vi "6.1.1.-Lógica Difusa Motor.vi"() -> (3 "Posicion":dbl(knob), 11 "Tensión":dbl(slide) scale=-12.0..12.0)   [LabVIEW 2020]
uses:
  <vilib>/addons/Fuzzy Logic/FL Fuzzy Controller (SISO).vi
  <vilib>/addons/Fuzzy Logic/NI_Fuzzy_Logic_API.lvlib
panel:
  out "XY Graph":cluster{i32[], dbl[]}(graph)
  out "Array":dbl[](array[numeric])
  in  "stop":bool
  in  "Set Point":dbl(slide) scale=0.0..360.0
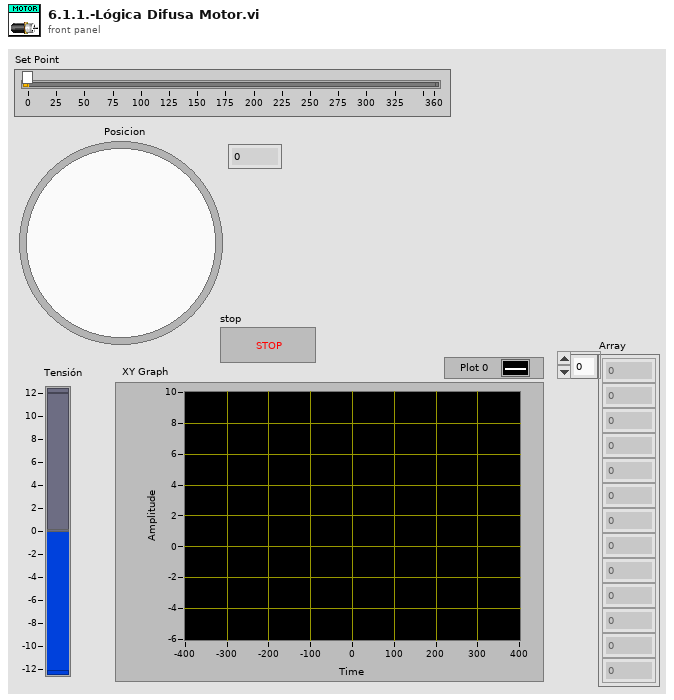
[diagram p1: front panel]
types:
  T1 = typedef "NI_Fuzzy_Logic_API.lvlib/FL System.ctl" = cluster{"input variables":T2[], "output variables":T2[], "rules":T5[], "defuzzification method":T11, "description":string, "user MF interpolating polynomials":T12[]}
  T2 = typedef "NI_Fuzzy_Logic_API.lvlib/FL Variable.ctl" = cluster{"name":string, "range":dbl[], "MFs":T3[]}
  T3 = typedef "NI_Fuzzy_Logic_API.lvlib/FL Membership Function.ctl" = cluster{"name":string, "shape":T4, "points":dbl[], "color":u32, "user-defined shape index":i32}
  T4 = typedef "NI_Fuzzy_Logic_API.lvlib/FL Membership Function Shape.ctl" = u16
  T5 = typedef "NI_Fuzzy_Logic_API.lvlib/FL Rule.ctl" = cluster{"antecedents":T6[], "antecedent connective":T8, "consequents":T9[], "consequent implication":T10, "degree of support":dbl}
  T6 = typedef "NI_Fuzzy_Logic_API.lvlib/FL Antecedent.ctl" = cluster{"Var Index":i32, "MF Index":i32, "Cond":T7}
  T7 = typedef "NI_Fuzzy_Logic_API.lvlib/FL Modifier.ctl" = u16
  T8 = typedef "NI_Fuzzy_Logic_API.lvlib/FL Antecedent Connective.ctl" = u16
  T9 = typedef "NI_Fuzzy_Logic_API.lvlib/FL Consequent.ctl" = cluster{"Var Index":i32, "MF Index":i32, "Cond":T7}
  T10 = typedef "NI_Fuzzy_Logic_API.lvlib/FL Consequent Implication.ctl" = u16
  T11 = typedef "NI_Fuzzy_Logic_API.lvlib/FL Defuzzification.ctl" = u16
  T12 = typedef "NI_Fuzzy_Logic_API.lvlib/FL Interpolating polynomials.ctl" = cluster{"X":dbl[], "Y":dbl[], "Y(x) coeff":dbl[][], "X(y) coeff":dbl[][], "Area(y) coeff":dbl[][], "coa_x(y) coeff":dbl[][]}
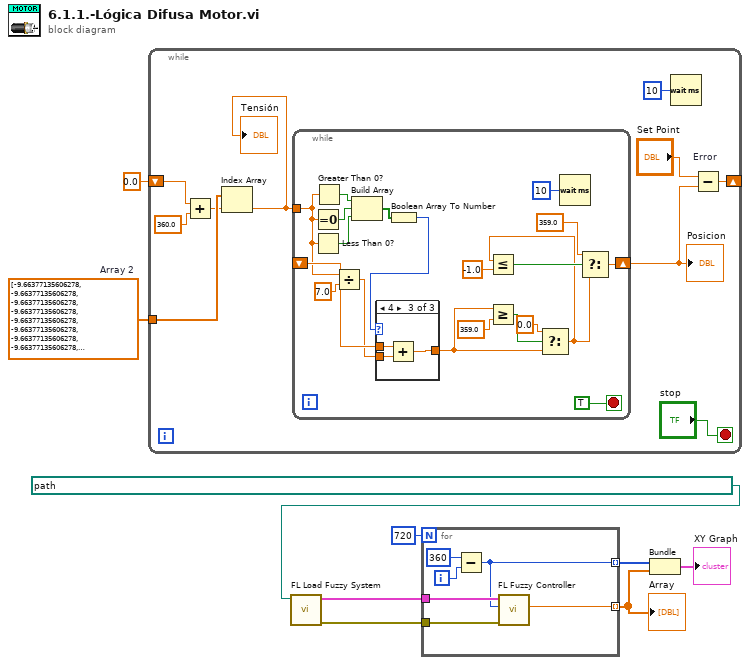
[diagram p0: block diagram]
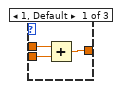
[diagram p2: hidden frame]
diagram:
  w1 = dbl[] [-9.66377135606278, -9.66377135606278, -9.66377135606278, -9.66377135606278, -9.66377135606278, -9.66377135606278, -9.66377135606278, -9.66377135606278, -9.66377135606278, -9.66377135606278, -9.66377135606278, -9.66377135606278, -9.66377135606278, -9.66377135606278, -9.66377135606278, -9.66377135606278, -9.66377135606278, -9.66377135606278, -9.66377135606278, -9.66377135606278, -9.66377135606278, -9.66377135606278, -9.66377135606278, -9.66377135606278, -9.66377135606278, -9.66377135606278, -9.66377135606278, -9.66377135606278, -9.66377135606278, -9.66377135606278, -9.66377135606278, -9.66377135606278, -9.66377135606278, -9.66377135606278, -9.66377135606278, -9.66377135606278, -9.66377135606278, -9.66377135606278, -9.66377135606278, -9.66377135606278, -9.66377135606278, -9.66377135606278, -9.66377135606278, -9.66377135606278, -9.66377135606278, -9.66377135606278, -9.66377135606278, -9.66377135606278, -9.66377135606278, -9.66377135606278, -9.66377135606278, -9.66377135606278, -9.66377135606278, -9.66377135606278, -9.66377135606278, -9.66377135606278, -9.66377135606278, -9.66377135606278, -9.66377135606278, -9.66377135606278, -9.66377135606278, -9.602567611575033, -9.541862924617375, -9.481651215975328, -9.421926504772852, -9.362682906491901, -9.303914631039657, -9.244328181919316, -9.187821091365203, -9.133216921575809, -9.079043687583988, -9.025296308026498, -8.971969781116245, -8.91905918309065, -8.866559666696107, -8.814466459707706, -8.76277486348314, -8.711480251549936, -8.66057806822514, -8.610063827266517, -8.559933110554525, -8.510181566804137, -8.46074884357682, -8.418094863909172, -8.375889018091348, -8.33385061736725, -8.291978667241288, -8.250272181077706, -8.208730180023073, -8.167351692929728, -8.126135756280064, -8.08458400446258, -8.042461828178011, -8.00057677537656, -7.95892684937627, -7.917510075849662, -7.876324502511783, -7.836119326659839, -7.79819112131189, -7.760440752628416, -7.722866972781734, -7.685468545591136, -7.648244246387266, -7.611192861878472, -7.574313190018964, -7.537604039878832, -7.5010443555021755, -7.464413266940578, -7.4279199209420534, -7.391563542041992, -7.355343360585824, -7.319258612674724, -7.285949116533284, -7.254699798339329, -7.223515170326685, -7.192395031827329, -7.161317190840123, -7.130325267582253, -7.099422687499635, -7.068609064812042, -7.037884015957109, -7.007247159574394, -6.976698116489636, -6.9462365096990695, -6.91586196435395, -6.88557410774515, -6.855372569287947, -6.8269062701543985, -6.7987291960853815, -6.77060930354623, -6.742546418650207, -6.714119548633666, -6.685283733960341, -6.656408950727237, -6.627522459838097, -6.598624254170943, -6.569714326598021, -6.540792669985794, -6.511859277194934, -6.482914141080324, -6.4539572544910335, -6.4255452155999135, -6.399570969318972, -6.373543875051162, -6.347463771343066, -6.321330496082931, -6.295143886497309, -6.268903779147681, -6.242610009927052, -6.216262414056531, -6.189701785954419, -6.162867037973021, -6.135932903288173, -6.10889882873411, -6.081764257032361, -6.054528626753464, -6.027768904888585, -6.0014956107977575, -5.976187022973889, -5.9510616641367875, -5.925862874705745, -5.900590332300716, -5.8752437126517645, -5.8498226895852135, -5.824326935009648, -5.79875611890179, -5.773109909292277, -5.747387972251279, -5.721574419432044, -5.695518359202395, -5.669362850943312, -5.644440395152999, -5.619727133509676, -5.594876515472104, -5.569887392708088, -5.544758604049223, -5.519973566001828, -5.495685899353129, -5.471282522457748, -5.446762606448659, -5.422125314523331, -5.397369801848523, -5.372495215463717, -5.347500694183157, -5.32238536849646, -5.29719932379442, -5.272328422653832, -5.247066777713917, -5.221525696016304, -5.195790676804522, -5.169859502762561, -5.143729922643894, -5.11739965061997, -5.0908663656136115, -5.064355820327918, -5.040639459585903, -5.016781897703681, -4.992781869903006, -4.968638096255104, -4.944349281453124, -4.920015121091849, -4.8956488914145195, -4.871089069614369, -4.846333339326462, -4.82137934708358, -4.796166136073796, -4.770627065319108, -4.744856356126937, -4.718850842712282, -4.692607301337395, -4.666122448979593, -4.666122448979593, -4.666122448979593, -4.666122448979593, -4.666122448979593, -4.666122448979593, -4.665974085361705, -4.665743113875069, -4.665511918544546, -4.6652804990445755, -4.665048855048962, -4.664823742717059, -4.664602732085556, -4.664381075696181, -4.664158770714593, -4.663935814289835, -4.663712203554218, -4.663487935623198, -4.663263007595254, -4.6630374165517505, -4.662811159556827, -4.662584233657263, -4.6623566358823485, -4.662128363243756, -4.661634601556013, -4.660440470721498, -4.65946207826866, -4.658503151845306, -4.657538463367321, -4.65656796074313, -4.655591591251354, -4.654609301531252, -4.65362103757302, -4.652626744707875, -4.651626367597976, -4.650619850226163, -4.649607135885501, -4.648588167168621, -4.647562885956887, -4.646531233409329, -4.645699289179396, -4.645668560719857, -4.645637574666107, -4.644900326948918, -4.644084328893788, -4.643260525293575, -4.642428803612462, -4.641589049140895, -4.640741144942827, -4.639884971801439, -4.639020408163266, -4.638147330080661, -4.637265611152561, -4.6363751224634795, -4.63547573252067, -4.634980573065503, -4.6348790662002655, -4.634776413157728, -4.63467259441436, -4.634567590000691, -4.6344613794885055, -4.633117424753972, -4.630697548591472, -4.628243632472906, -4.625754953059972, -4.623230766373886, -4.620670307053868, -4.618072787583446, -4.615437397482888, -4.612763302466092, -4.611980173972492, -4.6116221714488965, -4.611257874415769, -4.610887115392786, -4.610509720904837, -4.610125511211395, -4.609734300021062, -4.609335894190391, -4.608930093405926, -4.608227230255004, -4.606117170096181, -4.603963880942782, -4.601766020591362, -4.59952219069252, -4.597437413307896, -4.596803168782329, -4.59615429362253, -4.595490275676275, -4.594810578604951, -4.594114640438743, -4.593401872027007, -4.59267165537482, -4.591923341855887, -4.591156250290884, -4.590369664879315, -4.589562832971661, -4.588734962667249, -4.587885220221753, -4.582953994092828, -4.578969620421459, -4.5776863654930455, -4.57635787555434, -4.574981715877343, -4.573555273812931, -4.572075742236131, -4.570540101107925, -4.568945096898777, -4.567287219578867, -4.565562676832542, -4.563767365098355, -4.56189683696917, -4.559946264407187, -4.557910397133364, -4.555783515436167, -4.556357795824015, -4.557996462536207, -4.557859524402199, -4.555272430381818, -4.55254080072598, -4.549652175001101, -4.546592618109409, -4.543346495483677, -4.539896205864125, -4.5362218620166965, -4.532300907163601, -4.528107651499963, -4.523612708673419, -4.518782306096311, -4.514121022235627, -4.522404838921037, -4.531454066600123, -4.5413799277279185, -4.552316290754712, -4.564425742933649, -4.5765601265573705, -4.571554353636676, -4.565847618449445, -4.5592816017791105, -4.551646425441341, -4.542657803346746, -4.531920859947032, -2.8412145345943256, -1.8586055582642607, -1.3105503675740113, -0.9438025590367929, -0.7263196832917511, -0.5436229558527924, -0.39279477072002406, -0.25453229717396364, -0.1254630510224033, -0.0032653061224489225, 0.11542856078754267, 0.23448596162466043, 0.36026146399880266, 0.505482919821349, 0.6990563290491673, 0.9294868479576326, 1.2596860719252931, 1.745490004875671, 2.6779492284718756, 4.408352084087297, 4.4294699915894515, 4.447232589533868, 4.462380686729483, 4.475451960302868, 4.486846113150682, 4.496866463120682, 4.4971430280058735, 4.496761991162808, 4.496418528420111, 4.496107343147028, 4.495824089553391, 4.49556516848782, 4.501527471398613, 4.507290105392767, 4.512630505269966, 4.517593437287113, 4.522217555415241, 4.526536410103456, 4.530579263644331, 4.534371754059134, 4.537936439349421, 4.541293246532926, 4.544459844347256, 4.54745195434275, 4.545656747601667, 4.54041380076149, 4.537371917148686, 4.539768569280606, 4.54206793734138, 4.544275826884357, 4.546397590534008, 4.548438171310814, 4.55040214107641, 4.552293734728412, 4.5541168806831855, 4.555875228108365, 4.55757217130234, 4.559210871563488, 4.560794276845593, 4.56232513945654, 4.563806032023897, 4.566616955083656, 4.569872778163102, 4.571034448782529, 4.572164122324139, 4.573263102820957, 4.574332624395031, 4.575373855880468, 4.576387905084468, 4.577375822718878, 4.5783386060317275, 4.579277202165022, 4.580192511262647, 4.581085389349762, 4.5819566510030585, 4.58280707182942, 4.586544440917215, 4.590605875416383, 4.594584233192338, 4.598482037443076, 4.602301710211596, 4.603313068324277, 4.603737713561558, 4.604155170698017, 4.60456562071469, 4.604969238567555, 4.605366193436195, 4.605756648960234, 4.606140763464269, 4.606518690171904, 4.607106566234939, 4.608638568813411, 4.610148298461914, 4.611636237395654, 4.613102854009453, 4.614548603369336, 4.615973927683301, 4.617379256752266, 4.618765008402167, 4.619604156197825, 4.619815019662677, 4.620023241836633, 4.62022887203831, 4.620431958366067, 4.620632547735527, 4.621613091722679, 4.623394713631733, 4.625158689480138, 4.6269052801389075, 4.628634741362142, 4.630347323911888, 4.632043273679325, 4.633722831802477, 4.635386234780509, 4.637033714584735, 4.638665498766462, 4.640281810561773, 4.64174028064541, 4.641781680554135, 4.641822778772909, 4.642263480891475, 4.642803664208371, 4.643340505112752, 4.643874034530963, 4.644404283008992, 4.64493128071829, 4.645455057461499, 4.645975642678068, 4.646493065449769, 4.647007354506114, 4.647518538229667, 4.648026644661273, 4.648531701505186, 4.649033736134091, 4.64958211905478, 4.650561240765731, 4.651184327164498, 4.651671711480727, 4.65215765130222, 4.652642153041195, 4.6531252230719815, 4.653606867731285, 4.654087093318477, 4.6545659060958595, 4.655043312288944, 4.655519318086718, 4.655993929641916, 4.656467153071274, 4.656938994455811, 4.6574103226289765, 4.657881849775383, 4.658352461797464, 4.658822161356703, 4.659290951104269, 4.659591836734692, 4.659591836734692, 4.659591836734692, 4.659591836734692, 4.659591836734692, 4.659591836734692, 4.6871011742617235, 4.714346801030888, 4.741332490940301, 4.768061946220208, 4.794538799126206, 4.820571739024343, 4.846292764658939, 4.871821577045187, 4.8971603227770135, 4.922311116603319, 4.947356490730332, 4.972291000027044, 4.997065265437661, 5.021680826747202, 5.046139204075932, 5.070441898192287, 5.09605298275151, 5.121591977171418, 5.146947186381057, 5.172120587116747, 5.197114127867872, 5.221929729379619, 5.246569285145048, 5.270990638436955, 5.295138165843044, 5.320049569742689, 5.3449530275259525, 5.369747513222112, 5.39443374052673, 5.41901241691662, 5.4434842437174495, 5.467849916170432, 5.492110123498185, 5.516265548969698, 5.5415456380354335, 5.567640576779736, 5.593579086358581, 5.619362569167972, 5.6449924108904534, 5.670642948617669, 5.696827459698597, 5.722879291578579, 5.748513382367604, 5.774030295021378, 5.799461451247165, 5.824807282630946, 5.850068217867501, 5.875244682784568, 5.900337100366785, 5.925345890779369, 5.950271471391572, 5.975114256799896, 6.0000025894850495, 6.025327053898483, 6.051755029804096, 6.0792657049941665, 6.106708384921412, 6.134083321359879, 6.161390764842107, 6.188630964666791, 6.215716264834649, 6.242677495875661, 6.269594583190768, 6.296467635106326, 6.323296759594542, 6.350082064274923, 6.376823656415714, 6.403521642935329, 6.43017613040378, 6.45803782856668, 6.48615613150014, 6.514251557513243, 6.542324134513474, 6.570373890362939, 6.598400852878466, 6.6264050498316855, 6.654386508949136, 6.682345257912353, 6.71022618305554, 6.737706664141921, 6.765019827451426, 6.79237741199007, 6.819779526213886, 6.847689412406526, 6.878995274739651, 6.910403476232794, 6.941914519529056, 6.973528910568595, 7.00524715861572, 7.037069776286238, 7.068997279575053, 7.101030187884076, 7.133169024050376, 7.165414314374626, 7.197758487281166, 7.230109119421513, 7.262513502908877, 7.29497177181836, 7.328485166137082, 7.363411078717199, 7.398424415358849, 7.43352550472391, 7.46871467712376, 7.503992264529646, 7.538940662970389, 7.573996360751456, 7.609199775709396, 7.644551843488171, 7.6800535076503085, 7.7157057197608605, 7.751509439472416, 7.787465634611224, 7.823575281264357, 7.8640118836404245, 7.9061944956687045, 7.948631362712731, 7.9913247904983855, 8.034277112715566, 8.077490691443403, 8.1205654841291, 8.16361788617886, 8.206896551724139, 8.250403269168725, 8.29413984581379, 8.338108108108106, 8.382309901902335, 8.426747092707314, 8.471562085548374, 8.51994069003066, 8.56864055058746, 8.617690795575259, 8.667095220050884, 8.716857674076063, 8.766982063717574, 8.81747235206932, 8.868332560296848, 8.91956676870493, 8.971179117828783, 9.023173809549522, 9.075555108234491, 9.128327341903175, 9.181494903419251, 9.237994858309824, 9.300174198756533, 9.360232908953055, 9.42074890713025, 9.481727435943963, 9.543173818497884, 9.605093459892602, 9.667491848810528, 9.667491848810528, 9.667491848810528, 9.667491848810528, 9.667491848810528, 9.667491848810528, 9.667491848810528, 9.667491848810528, 9.667491848810528, 9.667491848810528, 9.667491848810528, 9.667491848810528, 9.667491848810528, 9.667491848810528, 9.667491848810528, 9.667491848810528, 9.667491848810528, 9.667491848810528, 9.667491848810528, 9.667491848810528, 9.667491848810528, 9.667491848810528, 9.667491848810528, 9.667491848810528, 9.667491848810528, 9.667491848810528, 9.667491848810528, 9.667491848810528, 9.667491848810528, 9.667491848810528, 9.667491848810528, 9.667491848810528, 9.667491848810528, 9.667491848810528, 9.667491848810528, 9.667491848810528, 9.667491848810528, 9.667491848810528, 9.667491848810528, 9.667491848810528, 9.667491848810528, 9.667491848810528, 9.667491848810528, 9.667491848810528, 9.667491848810528, 9.667491848810528, 9.667491848810528, 9.667491848810528, 9.667491848810528, 9.667491848810528, 9.667491848810528, 9.667491848810528, 9.667491848810528, 9.667491848810528, 9.667491848810528, 9.667491848810528, 9.667491848810528, 9.667491848810528, 9.667491848810528, 9.667491848810528]  # Array 2
  n1 = while {
    shift-right: [w15] -> _
    shift-left: 0.0 -> [w12]
    tunnel: w1 -> [w14]
    stop <- "stop" stop-if-true
    n2 = Add(x=w12, y=360.0) -> (x+y=w11:dbl)
    n3 = Index Array "Index Array"(array=w14, index=w11) -> (element=w10:dbl)
    "Tensión" <- w10
    n4 = while {
      shift-right: [w24] -> w19
      shift-left: _ -> [w33]
      tunnel: w10 -> [w21]
      stop <- TRUE stop-if-true
      n5 = Equal To 0?(x=w21) -> (x = 0?=w38:bool)
      n6 = Less Than 0?(x=w21) -> (x < 0?=w36:bool)
      n7 = Greater Than 0?(x=w21) -> (x > 0?=w37:bool)
      n8 = Divide(x=w21, y=7.0) -> (x/y=w23:dbl)
      n9 = Build Array "Build Array"(w37, w38, w36) -> (w35:bool[])
      n10 = Boolean Array To Number(Boolean array=w35) -> (number=w34:u32)
      n11 = case shown="4" w34 {
        tunnel: w33 -> [w42 w43 w46]
        tunnel: [w40 w43 w44] -> w29
        tunnel: w23 -> [w41 _ w45]
        frame 1, Default {
          n12 = Add(x=w42, y=w41) -> (x+y=w40:dbl)
        }
        frame 2 {
        }
        frame 4 {
          n13 = Add(x=w46, y=w45) -> (x+y=w44:dbl)
        }
      }
      n14 = Greater Or Equal?(x=w29, y=359.0) -> (x >= y?=w31:bool)
      n15 = Select(t=0.0, s=w31, f=w29) -> (s? t:f=w25:dbl)
      n16 = Less Or Equal?(x=w25, y=-1.0) -> (x <= y?=w27:bool)
      n17 = Wait (ms)(milliseconds to wait=u32 10) -> ()  [unwired: 1 out]
      n18 = Select(t=359.0, s=w27, f=w25) -> (s? t:f=w24:dbl)
    }
    "Posicion" <- w19
    n19 = Wait (ms)(milliseconds to wait=u32 10) -> ()  [unwired: 1 out]
    n20 = Subtract "Error"(x="Set Point", y=w19) -> (x-y=w15:dbl)
  }
  n21 = call <vilib>:"FL Load Fuzzy System.vi"("file path"=path "C:/Users/diego/OneDrive/Documents/Aprendiendo/LabVIEW/1.-Sistemas de Visión Artificial/6.1.0.-Modelo Lógica Difusa Motor.fs") -> ("error out"=w7:errorcluster, "fuzzy system out"=w8:T1)  [unwired: 9 in]
  n22 = for {
    N: 720 -> [_]
    tunnel: w8 -> [w52]
    tunnel: w7 -> [w51]
    tunnel: [w50] -> w4 mode=indexing
    tunnel: [w49] -> w3 mode=indexing
    i -> [w47]
    n23 = Subtract(x=u16 360 ("y"), y=w47) -> (x-y=w50:i32)
    n24 = call-poly <vilib>:"FL Fuzzy Controller.vi"("error in (no error)"=w51, "input value"=w50, "fuzzy system in"=w52) -> ("output value"=w49:dbl)  [unwired: 4 in, 4 out]
  }
  "Array" <- w3
  n25 = Bundle "Bundle"(w4, w3) -> (→"XY Graph":cluster{i32[], dbl[]})  [unwired: 1 in]
